vi "Initialize CAD.vi"(8 "error in (no error)":errorcluster, 9 "progress":refnum<vi>) -> (0 "error out":errorcluster, 1 "Success":bool)   [LabVIEW 2012, in "Design Server.lvlib"]
uses:
  Design Server.lvlib
  AutoCAD cmds.ctl
  Word cmd.ctl
  Mathcad15 cmds.ctl
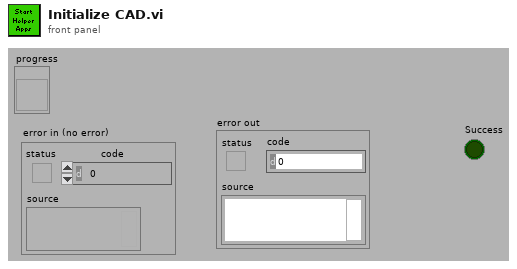
[diagram p1: front panel]
types:
  T1 = typedef "Design Server.lvlib/Mathcad15 cmds.ctl" = enum16{"Open Mathcad", "Execute Method", "Quit Mathcad"}
  T2 = typedef "Design Server.lvlib/Word cmd.ctl" = enum16{"Initialize", "Create Reports", "Quit"}
  T3 = typedef "Design Server.lvlib/AutoCAD cmds.ctl" = enum16{"Open AutoCAD", "Create Drawing", "Quit"}
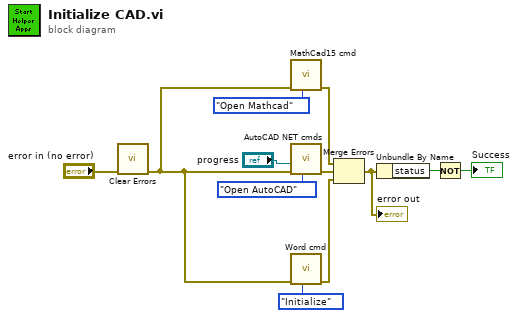
[diagram p0: block diagram]
diagram:
  n1 = call <vilib>:"Clear Errors.vi"("error in (no error)"="error in (no error)") -> ("error out"=w2:errorcluster)  [unwired: 6 in]
  n2 = call "MathCad15 cmd.vi"("Mathcad15 cmds"=Mathcad15_cmds."Open Mathcad", "error in"=w2) -> ("first error out"=w5:errorcluster)  [unwired: 7 in, 2 out]
  n3 = call "AutoCAD NET cmds.vi"("AutoCAD cmd"=AutoCAD_cmds."Open AutoCAD", "error in (no error)"=w2, "progress"="progress") -> ("error out"=w3:errorcluster)  [unwired: 7 in, 1 out]
  n4 = call "Word cmd.vi"("Word cmd"=Word_cmd."Initialize", "Error In (no error)"=w2) -> ("error out"=w4:errorcluster)  [unwired: 8 in, 1 out]
  n5 = Merge Errors(w5, w3, w4) -> (w10:errorcluster)
  "error out" <- w10
  n6 = Unbundle By Name(w10) -> ("status"=w11:bool)
  n7 = Not(x=w11) -> (.not. x?=→"Success":bool)
